vi "Ctrl Refnum to Value (Variant).vi"(13 "Ctl Refnum":refnum<vi>, 14 "Error In":errorcluster) -> (2 "Value":variant, 3 "Error Out":errorcluster)   [LabVIEW 2021, in "Variant.lvlib"]
uses:
  Variant.lvlib
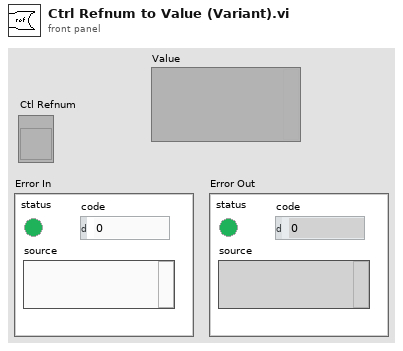
[diagram p1: front panel]
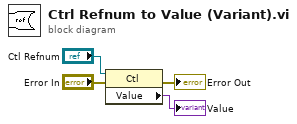
[diagram p0: block diagram]
diagram:
  n1 = property class="Ctl"(reference="Ctl Refnum", error in="Error In") -> (error out=→"Error Out":errorcluster, "Value"=→"Value":variant)  [unwired: 1 out]
